vi "Autonics Control.vi"() -> ()   [LabVIEW 2011]
uses:
  <vilib>/Instr/_visa.llb/VISA Configure Serial Port (Instr).vi
panel:
  in  "flow control (0:none)":u16(ring) items=["None", "XON/XOFF", "RTS/CTS", "XON/XOFF & RTS/CTS", "DTR/DSR", "XON/XOFF & DTR/DSR"]
  in  "stop bits (10: 1 bit)":u16(ring)=10 items=["1.0"=10, "1.5"=15, "2.0"=20]
  in  "Travel per Pulse (mm)":dbl=0.002
  in  "Speed (mm/s)":dbl=2.0
  out "Current  Position":dbl format="%#_4g"
  in  "Move Distance (mm)":dbl=1.0
  in  "Exit":bool
  in  "Stop":bool
  in  "Home":bool
  in  "Right":bool
  in  "Left":bool
  in  "Parity":dbl
  in  "Data bits":u16=8 min=5 max=8 step=1
  in  "Baud Rate":u32=57600
  in  "COM Port":refnum<visa-resource-name>="COM12"
  # "AUTONICS CONTROL"
  # "COM Setting"
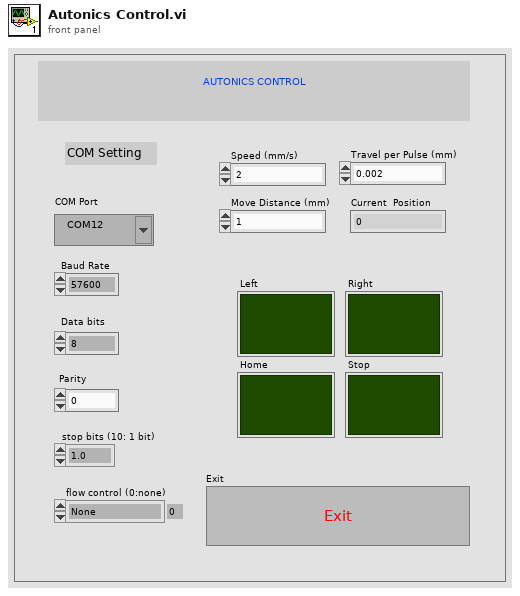
[diagram p1: front panel]
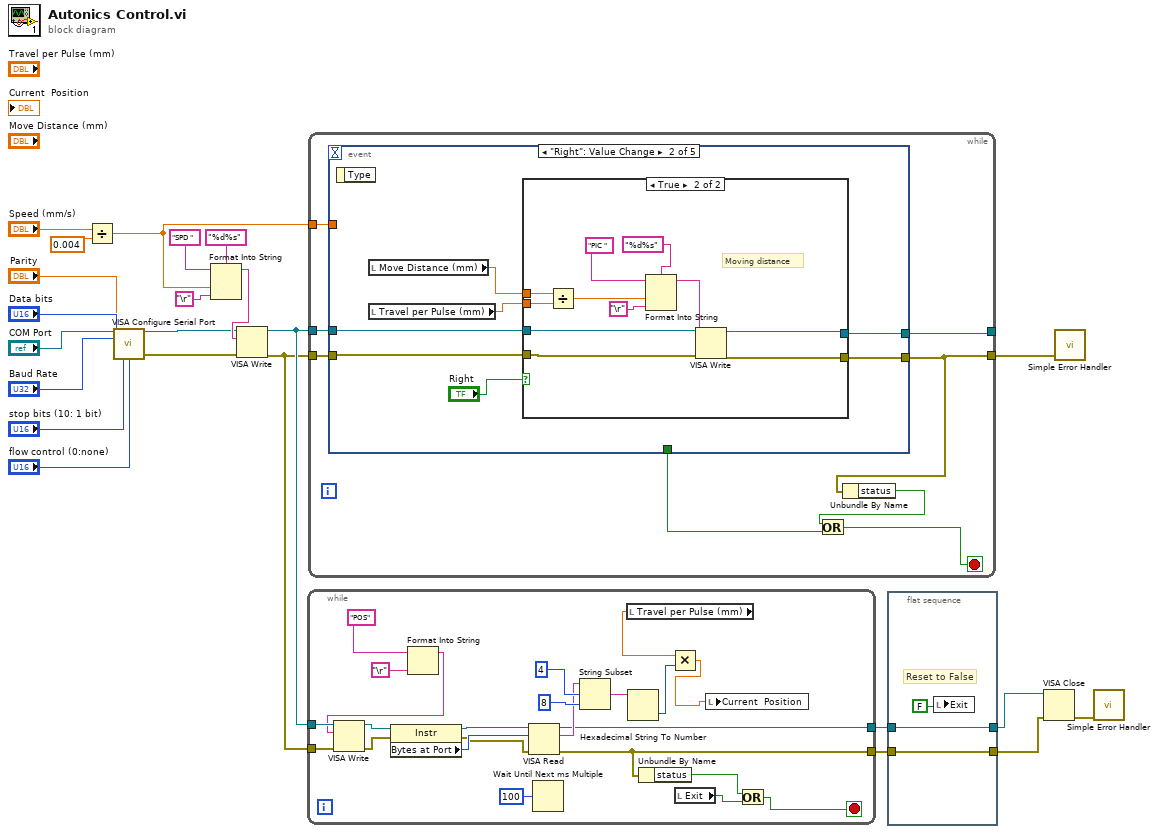
[diagram p0: block diagram]
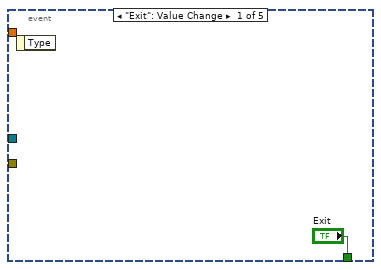
[diagram p2: hidden frame]
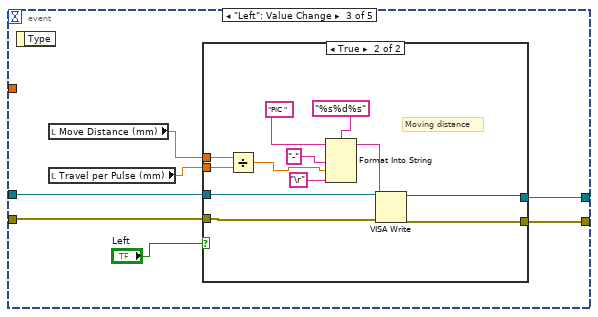
[diagram p4: hidden frame]
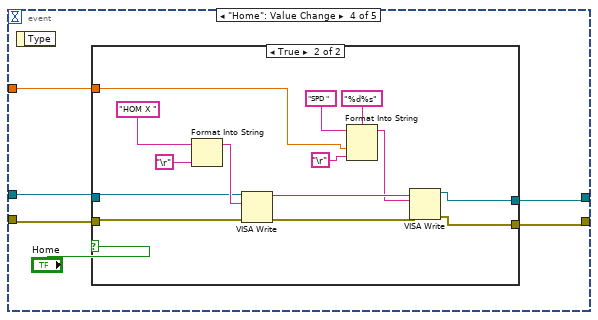
[diagram p6: hidden frame]
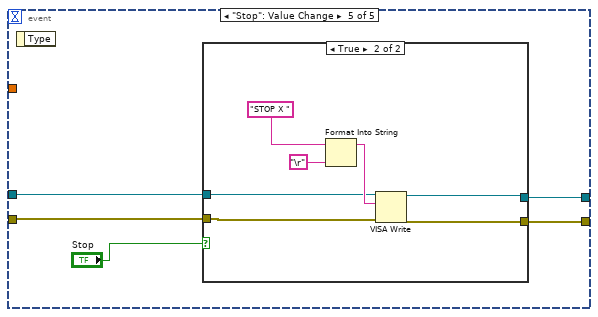
[diagram p8: hidden frame]
diagram:
  n1 = Divide(x="Speed (mm/s)", y=0.004) -> (x/y=w11:dbl)
  n2 = call-poly "VISA Configure Serial Port"("VISA resource name"="COM Port", "baud rate (9600)"="Baud Rate", "data bits (8)"="Data bits", "parity (0:none)"="Parity", "stop bits (10: 1 bit)"="stop bits (10: 1 bit)", "flow control (0:none)"="flow control (0:none)") -> ("VISA resource name out"=w7:refnum<visa-resource-name>, "error out"=w6:errorcluster)  [unwired: 8 in]
  n3 = Format Into String(format string="%d%s", initial string="SPD " ("string"), w11, "\r") -> (resulting string=w15:string)  [unwired: 1 in, 1 out]
  n4 = VISA Write(VISA resource name=w7, write buffer=w15, error in (no error)=w6) -> (VISA resource name out=w9:refnum<visa-resource-name>, error out=w8:errorcluster)  [unwired: 1 out]
  n5 = while {
    tunnel: w9 -> [w32]
    tunnel: w8 -> [w31]
    tunnel: [w28] -> w5
    tunnel: [w26] -> w4
    stop <- w24 stop-if-true
    n6 = Format Into String(initial string="POS" ("string"), "\r") -> (resulting string=w30:string)  [unwired: 2 in, 1 out]
    n7 = VISA Write(VISA resource name=w32, write buffer=w30, error in (no error)=w31) -> (VISA resource name out=w40:refnum<visa-resource-name>, error out=w39:errorcluster)  [unwired: 1 out]
    n8 = property class="Instr"(reference=w40, error in=w39) -> (reference out=w45:refnum<visa-resource-name>, error out=w43:errorcluster, "Bytes at Port"=w44:u32)
    n9 = VISA Read(VISA resource name=w45, byte count=w44, error in (no error)=w43) -> (VISA resource name out=w28:refnum<visa-resource-name>, read buffer=w29:string, error out=w26:errorcluster)  [unwired: 1 out]
    n10 = Wait Until Next ms Multiple(millisecond multiple=u32 100) -> ()  [unwired: 1 out]
    n11 = String Subset(string=w29, offset (0)=4, length (rest)=8 ("length (rest)")) -> (substring=w36:string)
    n12 = local read "Travel per Pulse (mm)"() -> (w33:dbl)
    n13 = Hexadecimal String To Number(string=w36) -> (number=w35:u32)  [unwired: 2 in, 1 out]
    n14 = Unbundle By Name(w26) -> ("status"=w25:bool)
    n15 = Multiply(x=w33, y=w35) -> (x*y=w34:dbl)
    n16 = local read "Exit"() -> (w27:bool)
    n17 = local write "Current  Position"(w34) -> ()
    n18 = Or(x=w25, y=w27) -> (x .or. y?=w24:bool)
  }
  n19 = while {
    tunnel: w9 -> [w53]
    tunnel: w8 -> [w52]
    tunnel: [w54] -> _
    tunnel: [w48] -> w1
    tunnel: w11 -> [w47]
    stop <- w49 stop-if-true
    n20 = event shown="[1] \"Right\": Value Change" {
      selector: _ -> [_ _ _ _ _]
      dyn-events: _ -> [_ _ _ _ _]
      timeout: _ -> [_ _ _ _ _]
      tunnel: w53 -> [_ w60 w80 w102 w121]
      tunnel: w52 -> [_ w59 w79 w101 w120]
      tunnel: [_ w62 w82 w99 w123] -> w54
      tunnel: [_ w61 w81 w98 w122] -> w48
      tunnel: ["Exit" _ _ _ _] -> w50
      tunnel: w47 -> [_ _ _ w97 _]
      event "Exit": Value Change {
        n21 = event-data() -> ()  [unwired: 1 in, 1 out]
      }
      event "Right": Value Change {
        n22 = event-data() -> ()  [unwired: 1 in, 1 out]
        n23 = local read "Move Distance (mm)"() -> (w56:dbl)
        n24 = local read "Travel per Pulse (mm)"() -> (w57:dbl)
        n25 = case shown="True" "Right" {
          tunnel: [w64 w71] -> w62
          tunnel: [w63 w70] -> w61
          tunnel: w60 -> [w64 w66]
          tunnel: w59 -> [w63 w65]
          tunnel: w57 -> [_ w73]
          tunnel: w56 -> [_ w72]
          frame False {
          }
          frame True {
            # "Moving distance"
            n26 = Divide(x=w72, y=w73) -> (x/y=w74:dbl)
            n27 = Format Into String(format string="%d%s", initial string="PIC " ("string"), w74, "\r") -> (resulting string=w67:string)  [unwired: 1 in, 1 out]
            n28 = VISA Write(VISA resource name=w66, write buffer=w67, error in (no error)=w65) -> (VISA resource name out=w71:refnum<visa-resource-name>, error out=w70:errorcluster)  [unwired: 1 out]
          }
        }
      }
      event "Left": Value Change {
        n29 = event-data() -> ()  [unwired: 1 in, 1 out]
        n30 = local read "Move Distance (mm)"() -> (w77:dbl)
        n31 = local read "Travel per Pulse (mm)"() -> (w78:dbl)
        n32 = case shown="True" "Left" {
          tunnel: [w84 w93] -> w82
          tunnel: [w83 w92] -> w81
          tunnel: w80 -> [w84 w89]
          tunnel: w79 -> [w83 w88]
          tunnel: w78 -> [_ w95]
          tunnel: w77 -> [_ w94]
          frame False {
          }
          frame True {
            # "Moving distance"
            n33 = Divide(x=w94, y=w95) -> (x/y=w87:dbl)
            n34 = Format Into String(format string="%s%d%s", initial string="PIC " ("string"), "-" ("input 1"), w87, "\r") -> (resulting string=w90:string)  [unwired: 1 in, 1 out]
            n35 = VISA Write(VISA resource name=w89, write buffer=w90, error in (no error)=w88) -> (VISA resource name out=w93:refnum<visa-resource-name>, error out=w92:errorcluster)  [unwired: 1 out]
          }
        }
      }
      event "Home": Value Change {
        n36 = event-data() -> ()  [unwired: 1 in, 1 out]
        n37 = case shown="True" "Home" {
          tunnel: [w104 w112] -> w99
          tunnel: [w103 w110] -> w98
          tunnel: w102 -> [w104 w116]
          tunnel: w101 -> [w103 w115]
          tunnel: w97 -> [_ w105]
          frame False {
          }
          frame True {
            n38 = Format Into String(initial string="HOM X " ("string"), "\r") -> (resulting string=w117:string)  [unwired: 2 in, 1 out]
            n39 = VISA Write(VISA resource name=w116, write buffer=w117, error in (no error)=w115) -> (VISA resource name out=w113:refnum<visa-resource-name>, error out=w111:errorcluster)  [unwired: 1 out]
            n40 = Format Into String(format string="%d%s", initial string="SPD " ("string"), w105, "\r") -> (resulting string=w106:string)  [unwired: 1 in, 1 out]
            n41 = VISA Write(VISA resource name=w113, write buffer=w106, error in (no error)=w111) -> (VISA resource name out=w112:refnum<visa-resource-name>, error out=w110:errorcluster)  [unwired: 1 out]
          }
        }
      }
      event "Stop": Value Change {
        n42 = event-data() -> ()  [unwired: 1 in, 1 out]
        n43 = case shown="True" "Stop" {
          tunnel: [w125 w132] -> w123
          tunnel: [w124 w131] -> w122
          tunnel: w121 -> [w125 w128]
          tunnel: w120 -> [w124 w127]
          frame False {
          }
          frame True {
            n44 = Format Into String(initial string="STOP X " ("string"), "\r") -> (resulting string=w129:string)  [unwired: 2 in, 1 out]
            n45 = VISA Write(VISA resource name=w128, write buffer=w129, error in (no error)=w127) -> (VISA resource name out=w132:refnum<visa-resource-name>, error out=w131:errorcluster)  [unwired: 1 out]
          }
        }
      }
    }
    n46 = Unbundle By Name(w48) -> ("status"=w51:bool)
    n47 = Or(x=w51, y=w50) -> (x .or. y?=w49:bool)
  }
  n48 = flat-sequence {
    tunnel: w5 -> [w134]
    tunnel: w4 -> [w133]
    tunnel: [w134] -> w3
    tunnel: [w133] -> w2
    frame #0 {
      # "Reset to False"
      n49 = local write "Exit"(FALSE) -> ()
    }
  }
  n50 = VISA Close(VISA resource name=w3, error in (no error)=w2) -> (error out=w19:errorcluster)
  n51 = call <vilib>:"Simple Error Handler.vi"("error in (no error)"=w1) -> ()  [unwired: 4 in, 5 out]
  n52 = call <vilib>:"Simple Error Handler.vi"("error in (no error)"=w19) -> ()  [unwired: 4 in, 5 out]
